vi "Asynch Simple UE9.vi"() -> ()   [LabVIEW 2021]
panel:
  out "Actual Baud Rate":dbl
  out "BaudFactor":i32
  in  "Desired Baud Rate":i32=9600
  out "Bytes in Read Buffer before read":i32
  in  "# Bytes To Write":i32=4 min=1 max=50
  out "U8 Array Read":u8[](array[numeric])=[99, 99, 99, 99, 99, 99, 99, 99, 99, 99, 99, 99, 99, 99, 99, 99, 99, 99, 99, 99, 99, 99, 99, 99, 99, 99, 99, 99, 99, 99, 99, 99]
  in  "U8 Array Write":u8[](array[numeric])=[170, 240, 170, 240]
  out "Error Message":string
  out "error out":errorcluster
  # "You can short TX to RX for loopback testing.\n\nTX       DB37-Pin2 on UE9\nRX      DB37-Pin20 on UE9\n\nThis simple VI simply does a write, waits 1 second, then returns whatever was read in that time.\nIf you short TX to RX, then you will read back the same bytes that you write."
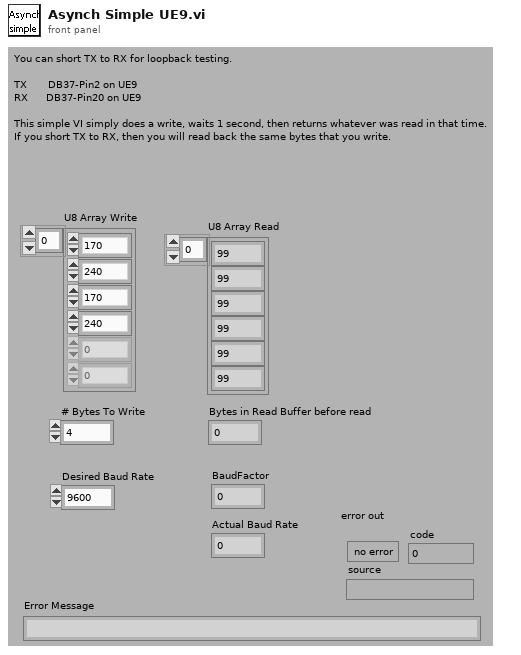
[diagram p1: front panel]
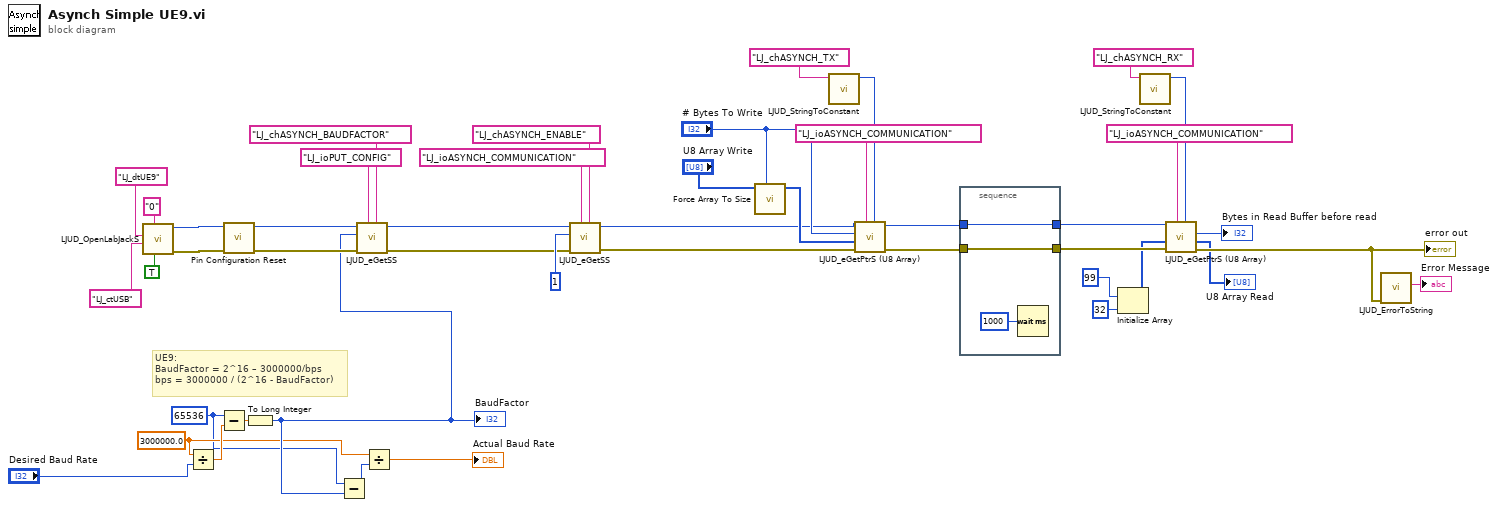
[diagram p0: block diagram]
diagram:
  w3 = 65536 ("x")
  w4 = 3000000.0 ("x")
  # "UE9:\nBaudFactor = 2^16 – 3000000/bps\nbps = 3000000 / (2^16 - BaudFactor)"
  n1 = call "LJUD_OpenLabJackS.vi"("FirstFound"=TRUE, "Address"="0", "ConnectionType"="LJ_ctUSB", "DeviceType"="LJ_dtUE9") -> ("error out"=w38:errorcluster, "Handle"=w37:i32)  [unwired: 5 in, 1 out]
  n2 = Divide(x=w4, y="Desired Baud Rate") -> (x/y=w7:dbl)
  n3 = Subtract(x=w3, y=w7) -> (x-y=w6:dbl)
  n4 = call "Pin Configuration Reset.vi"("error in"=w38, "Handle In"=w37) -> ("error out"=w40:errorcluster, "Handle Out"=w39:i32)  [unwired: 8 in]
  n5 = To Long Integer(number=w6) -> (32bit integer=w9:i32)
  "BaudFactor" <- w9
  n6 = Subtract(x=w3, y=w9) -> (x-y=w5:i32)
  n7 = call "LJUD_eGetSS.vi"("Channel"="LJ_chASYNCH_BAUDFACTOR", "IOType"="LJ_ioPUT_CONFIG", "error in"=w40, "Value Write"=w9, "Handle In"=w39) -> ("error out"=w30:errorcluster, "Handle Out"=w29:i32)  [unwired: 4 in, 1 out]
  n8 = Divide(x=w4, y=w5) -> (x/y=→"Actual Baud Rate":dbl)
  n9 = call "LJUD_eGetSS.vi"("Channel"="LJ_chASYNCH_ENABLE", "IOType"="LJ_ioASYNCH_COMMUNICATION", "error in"=w30, "Value Write"=1 ("Value"), "Handle In"=w29) -> ("error out"=w19:errorcluster, "Handle Out"=w18:i32)  [unwired: 4 in, 1 out]
  n10 = call "Force Array To Size.vi"("# Elements"="# Bytes To Write", "I32 Array In"="U8 Array Write") -> ("I32 Array Out"=w41:i32[])  [unwired: 6 in, 3 out]
  n11 = call "LJUD_StringToConstant.vi"("String"="LJ_chASYNCH_TX" ("Channel")) -> ("Constant Number"=w25:i32)  [unwired: 9 in, 1 out]
  n12 = call "LJUD_eGetPtrS (U8 Array).vi"("Channel"=w25, "IOType"="LJ_ioASYNCH_COMMUNICATION", "error in"=w19, "U8 Array Write"=w41, "Value"="# Bytes To Write", "Handle In"=w18) -> ("error out"=w20:errorcluster, "Handle Out"=w17:i32)  [unwired: 2 in, 2 out]
  n13 = stacked-sequence {
    tunnel: [w48] -> w15
    tunnel: w20 -> [w48]
    tunnel: [w47] -> w16
    tunnel: w17 -> [w47]
    frame #0 {
      n14 = Wait (ms)(milliseconds to wait=u32 1000) -> ()  [unwired: 1 out]
    }
  }
  n15 = Initialize Array(u8 99 ("Element Data"), 32 ("Dimension Size")) -> (w14:u8[])
  n16 = call "LJUD_StringToConstant.vi"("String"="LJ_chASYNCH_RX" ("Channel")) -> ("Constant Number"=w24:i32)  [unwired: 9 in, 1 out]
  n17 = call "LJUD_eGetPtrS (U8 Array).vi"("Channel"=w24, "IOType"="LJ_ioASYNCH_COMMUNICATION", "error in"=w15, "U8 Array Write"=w14, "Handle In"=w16) -> ("error out"=w22:errorcluster, "U8 Array Read"=→"U8 Array Read":u8[], "Value"=→"Bytes in Read Buffer before read":i32)  [unwired: 3 in, 1 out]
  "error out" <- w22
  n18 = call "LJUD_ErrorToString.vi"("error in"=w22) -> ("String"=→"Error Message":string)  [unwired: 10 in]
